vi "Find Frame Sink Terminal (by Name).vi"(8 "error in (no error)":errorcluster, 9 "Frame Name":string, 10 "Terminal Name":string, 11 "CaseStructure in":refnum<vi>) -> (0 "error IO":errorcluster, 1 "Found ?":bool, 2 "Terminal ref":refnum<vi>, 3 "CaseStructure out":refnum<vi>)   [LabVIEW 2019, in "gRPC Template Creation Utility.lvlib"]
uses:
  gRPC Template Creation Utility.lvlib
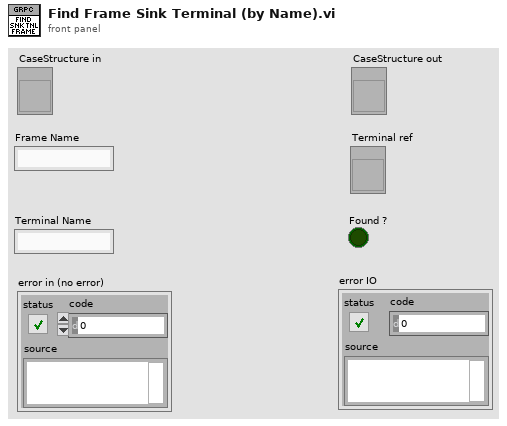
[diagram p1: front panel]
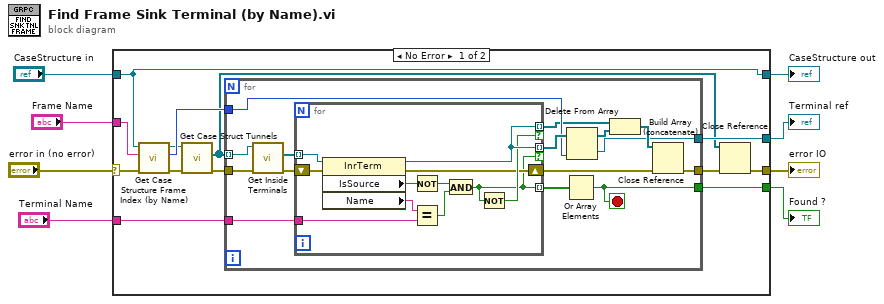
[diagram p0: block diagram]
diagram:
  n1 = case shown="No Error" "error in (no error)" {
    selector: "error in (no error)" -> [w15 w49]
    tunnel: "Terminal Name" -> [w21 _]
    tunnel: "Frame Name" -> [w17 _]
    tunnel: "CaseStructure in" -> [w12 w48]
    tunnel: [w14 _] -> w3
    tunnel: [w13 _] -> w2
    tunnel: [w12 w48] -> w4
    tunnel: [w9 w49] -> w1
    frame No Error {
      n2 = call "Get Case Structure Frame Index (by Name).vi"("error in (no error)"=w15, "element"=w17, "CaseStructure in"=w12) -> ("error out"=w19:errorcluster, "Frame Index"=w20:i32, "CaseStructure out"=w18:refnum<vi>)  [unwired: 5 in, 1 out]
      n3 = call "Get Case Struct Tunnels.vi"("Error In"=w19, "Case Structure in"=w18) -> ("Error Out"=w16:errorcluster, "Tunnels[]"=w10:refnum<vi>[])  [unwired: 7 in, 1 out]
      n4 = for {
        tunnel: w16 -> [w36]
        tunnel: w10 -> [w35] mode=indexing
        tunnel: w20 -> [w30]
        tunnel: w21 -> [w34]
        tunnel: [w26] -> w14
        tunnel: [w24] -> w13
        tunnel: [w22] -> w11
        stop <- w24 stop-if-true
        n5 = call "Get Inside Terminals.vi"("Error In"=w36, "Tunnel in"=w35) -> ("Error Out"=w33:errorcluster, "InsideTerms[]"=w32:refnum<vi>[])  [unwired: 7 in, 1 out]
        n6 = for {
          tunnel: w32 -> [w47] mode=indexing
          tunnel: w34 -> [w46]
          tunnel: [w42] -> w31 mode=indexing if=w38
          tunnel: [w42] -> w29 mode=indexing if=w41
          tunnel: [w38] -> w25 mode=indexing
          shift-right: [w39] -> w23
          shift-left: w33 -> [w43]
          n7 = property class="InrTerm"(reference=w47, error in=w43) -> (reference out=w42:refnum<vi>, error out=w39:errorcluster, "IsSource"=w44:bool, "Name"=w45:string)
          n8 = Not(x=w44) -> (.not. x?=w37:bool)
          n9 = Equal?(x=w45, y=w46) -> (x = y?=w40:bool)
          n10 = And(x=w37, y=w40) -> (x .and. y?=w38:bool)
          n11 = Not(x=w38) -> (.not. x?=w41:bool)
        }
        n12 = Or Array Elements(Boolean array=w25) -> (logical OR=w24:bool)
        n13 = Delete From Array(array=w31, index=w30) -> (deleted portion=w26:refnum<vi>, array with subset deleted=w28:refnum<vi>[])  [unwired: 1 in]
        n14 = Build Array (concatenate)(w29, w28) -> (w27:refnum<vi>[])
        n15 = Close Reference(reference=w27, error in (no error)=w23) -> (error out=w22:errorcluster)
      }
      n16 = Close Reference(reference=w10, error in (no error)=w11) -> (error out=w9:errorcluster)
    }
    frame Error {
    }
  }
  "CaseStructure out" <- w4
  "Terminal ref" <- w3
  "Found ?" <- w2
  "error IO" <- w1
